vi "Robot Global Data.vi"() -> ()   [LabVIEW 2025]
doc: "This global VI can contain as many global variables as you need. To create a global variable, place a control on the panel, give it a good name. To read or write to it from a VI, drag the icon to the diagram of that VI. You can also drag from the project. Click on the node to change which global you access. You shouldn't have multiple locations writing to a global or it will cause a race-condition."
uses:
  <vilib>/Rock Robotics/WPI/Camera/WPI_CameraImageSize.ctl
  <vilib>/Rock Robotics/WPI/DriverStation/WPI_DriverStationRobotMode2.ctl
  Drive Conditions.ctl
  Drive/Implementation/Drive Setpoints.ctl
  Drive/Implementation/Drive Operations.ctl
  swerve-template/Type Definitions/Data/Robot Velocities.ctl
  Drive/Implementation/Auto Data.ctl
  <vilib>/Rock Robotics/WPI/Framework/Command Status Info.ctl
  <vilib>/Rock Robotics/WPI/Framework/Completion Status.ctl
  <vilib>/Rock Robotics/WPI/Framework/Completion Notifier.ctl
  swerve-template/Type Definitions/Data/Pod Positions.ctl
  <vilib>/Rock Robotics/WPI/MotorControl/WPI_MotorControlDeviceRef.ctl
  <vilib>/Rock Robotics/WPI/MotorControl/WPI_MotorControlType.ctl
  <vilib>/Rock Robotics/SystemInterfaces/DIO/FPGA_DIOPWMChannel.ctl
  <vilib>/Rock Robotics/WPI/PWM/WPI_PWMDeadband.ctl
  <vilib>/Rock Robotics/SystemInterfaces/DIO/FPGA_DIOChannel.ctl
  Shooter/Implementation/Shooter Modes.ctl
panel:
  in  "Using Front LL4":bool
  in  "Shooter Modes":T1=enum."Idle"
  in  "Limelight Pose":cluster{"X":dbl, "Y":dbl}
  in  "Interp Flywheel":dbl
  in  "Interp Hood":dbl
  in  "Fire":bool
  in  "Robot Velocities":T2
  in  "Time in Flight":dbl
  in  "Kicker Speed":dbl
  in  "Flywheel Speed":dbl
  in  "Hood Setpoint":dbl
  in  "Insta360 Robot Pose":cluster{"X":dbl, "Y":dbl}
  in  "Auto Pickup Done?":bool
  in  "Align Button Pressed":bool
  in  "Ball Info":T3(array[cluster])
  in  "Dist to hub":dbl
  in  "IMU":dbl
  in  "Motor Data":T4[](array[typedef])
  in  "Pod Radius":dbl=0.9375
  out "Pod Locations":T9 {"Right Back Position" format="%.2f"; "Right Front Position" format="%.2f"; "Left Back Position" format="%.2f"; "Left Front Position" format="%.2f"}
  out "Drive Controller Data":T16
  in  "Auto Done?":bool
  in  "Drive Conditions":T17
  in  "Robot Mode":T18
  in  "image size":T19=enum."320x240"
  in  "Enable Vision":bool
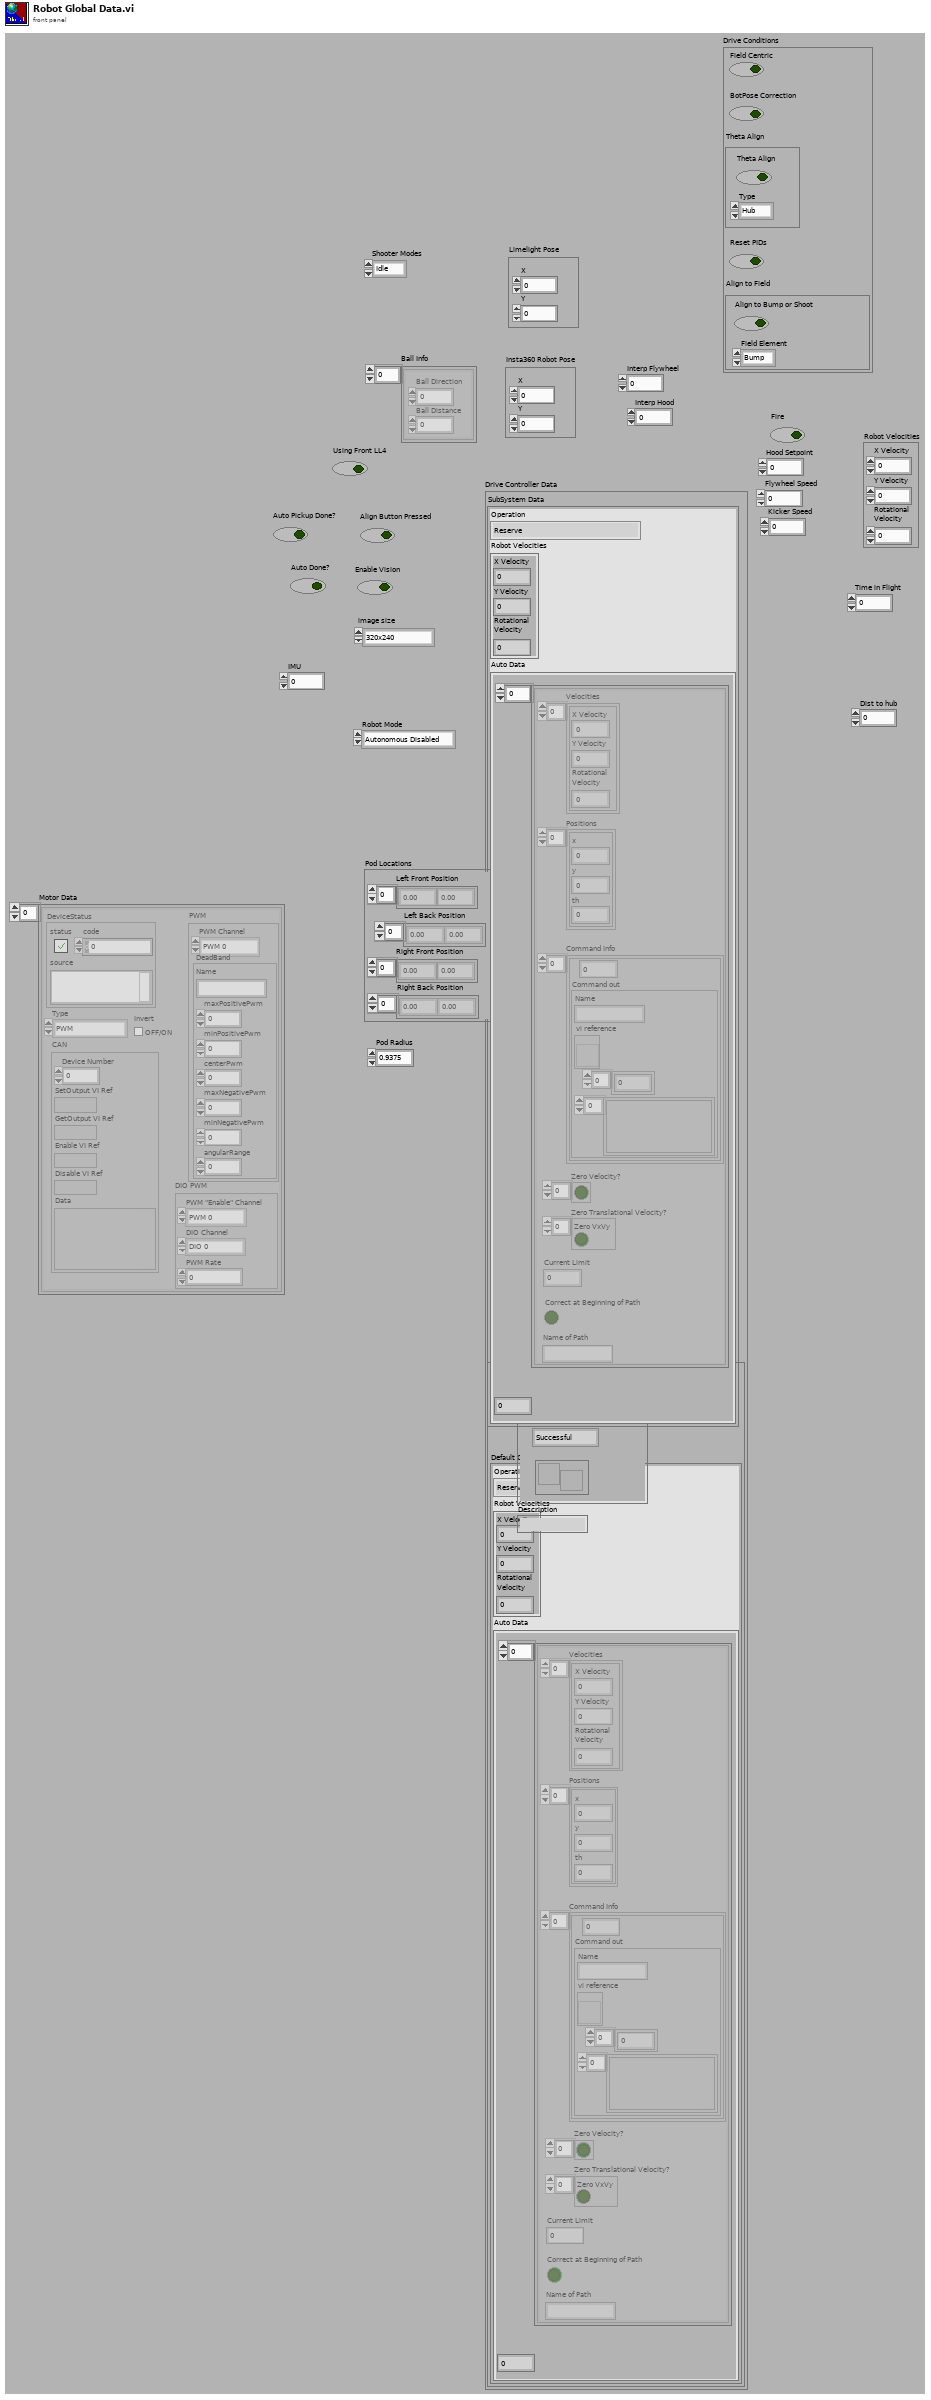
[diagram p1: front panel]
types:
  T1 = typedef "Shooter Modes.ctl" = enum16{"C to A Close", "C to A Far", "A to A", "Tower", "Interp", "Idle"}
  T2 = typedef "Robot Velocities.ctl" = cluster{"X Velocity":dbl, "Y Velocity":dbl, "Rotational \nVelocity":dbl}
  T3 = cluster{"Ball Direction":dbl, "Ball Distance":dbl}[]
  T4 = typedef "WPI_MotorControlDeviceRef.ctl" = cluster{"DeviceStatus":errorcluster, "Type":T5, "PWM":cluster{"PWM Channel":T6, "DeadBand":T7}, "CAN":cluster{"Device Number":u8, "SetOutput VI Ref":variant, "GetOutput VI Ref":variant, "Enable VI Ref":variant, "Disable VI Ref":variant, "Data":variant}, "Invert":bool, "DIO PWM":cluster{"PWM \"Enable\" Channel":T6, "DIOChannel":T8, "PWM Rate":dbl}}
  T5 = typedef "WPI_MotorControlType.ctl" = enum16{"PWM", "CAN", "DIO PWM"}
  T6 = typedef "FPGA_DIOPWMChannel.ctl" = enum8{"PWM 0", "PWM 1", "PWM 2", "PWM 3", "PWM 4", "PWM 5", "PWM 6", "PWM 7", "PWM 8", "PWM 9", "PWM MXP 0", "PWM MXP 1", "PWM MXP 2", "PWM MXP 3", "PWM MXP 4", "PWM MXP 5", "PWM MXP 6", "PWM MXP 7", "PWM MXP 8", "PWM MXP 9", "Invalid"}
  T7 = typedef "WPI_PWMDeadband.ctl" = cluster{"Name":string, "maxPositivePwm":i32, "minPositivePwm":i32, "centerPwm":i32, "maxNegativePwm":i32, "minNegativePwm":i32, "angularRange":u16}
  T8 = typedef "FPGA_DIOChannel.ctl" = enum8{"DIO 0", "DIO 1", "DIO 2", "DIO 3", "DIO 4", "DIO 5", "DIO 6", "DIO 7", "DIO 8", "DIO 9", "DIO MXP 0", "DIO MXP 1", "DIO MXP 2", "DIO MXP 3", "DIO MXP 4", "DIO MXP 5", "DIO MXP 6", "DIO MXP 7", "DIO MXP 8", "DIO MXP 9", "DIO MXP 10", "DIO MXP 11", "DIO MXP 12", "DIO MXP 13", "DIO MXP 14", "DIO MXP 15", "SPI Port CS1", "SPI Port CS2", "SPI Port CS3", "SPI Port MISO", "SPI Port MOSI", "Invalid"}
  T9 = typedef "Pod Positions.ctl" = cluster{"Left Front Position":dbl[], "Left Back Position":dbl[], "Right Front Position":dbl[], "Right Back Position":dbl[]}
  T10 = typedef "Drive Setpoints.ctl" = cluster{"Operation":T11, "Robot Velocities":T2, "Auto Data":T12}
  T11 = typedef "Drive Operations.ctl" = enum16{"Reserve", "Read Current", "Immediate", "Calibrate", "Auto", "Auto Pickup"}
  T12 = typedef "Auto Data.ctl" = cluster{"Auto Data":cluster{"Velocities":T2[], "Positions":cluster{"x":dbl, "y":dbl, "th":dbl}[], "Command Info":cluster{dbl, "Command out":cluster{"Name":string, "vi reference":refnum<vi>, i32[], variant[]}}[], "Zero Velocity?":bool[], "Zero Translational Velocity?":bool[], "Current Limit":dbl, "Correct at Beginning of Path":bool, "Name of Path":string}[], "Number of Remaining Auto Paths":dbl}
  T13 = typedef "Command Status Info.ctl" = cluster{"Name":string, "Status":T14, "notifier out":T15}
  T14 = typedef "Completion Status.ctl" = enum16{"Successful", "Aborted", "Incomplete"}
  T15 = typedef "Completion Notifier.ctl" = refnum<notifier>
  T16 = cluster{"SubSystem Data":T10, cluster{"Start Time (ms)":u32, "Iterations":i32}, cluster{"Command Info":T13, "Description":string, "Default Command":T10, "queue out":refnum<queue>, "Subsystem Name":string}}
  T17 = typedef "Drive Conditions.ctl" = cluster{"Field Centric":bool, "BotPose Correction":bool, "Theta Align":cluster{"Theta Align":bool, "Type":enum16{"Hub", "Corner of Field"}}, "Reset PIDs":bool, "Align to Field":cluster{"Align to Bump or Shoot":bool, "Field Element":enum16{"Bump", "Shooter Shot", "Trench"}}}
  T18 = typedef "WPI_DriverStationRobotMode2.ctl" = enum16{"Autonomous Disabled", "Autonomous Enabled", "Teleop Disabled", "Teleop Enabled", "Disconnected", "Finish", "Test Disabled", "Test Enabled", "Emergency Stopped"}
  T19 = typedef "WPI_CameraImageSize.ctl" = enum16{"640x480", "320x240", "160x120", "Custom"}
diagram:
